vi "sendErrorExplanation.vi"(8 "error in (no error)":errorcluster, 11 "TcpServerBase in":refnum<class "TcpServerBase.lvclass">) -> (0 "error out":errorcluster, 3 "TcpServerBase out":refnum<class "TcpServerBase.lvclass">)   [LabVIEW 2018, in "TcpServerBase.lvclass"]
doc: "Send a generic user event to the Component with the explanation of the error."
uses:
  TcpServerBase.lvclass
  TcpServerCmd/typedef/connStatusCluster.ctl
  <vilib>/Utility/error.llb/DialogType.ctl
  TcpServerBase.lvclass/TcpServerBase.ctl
  TcpServerCmd/TcpServerCmd.lvclass
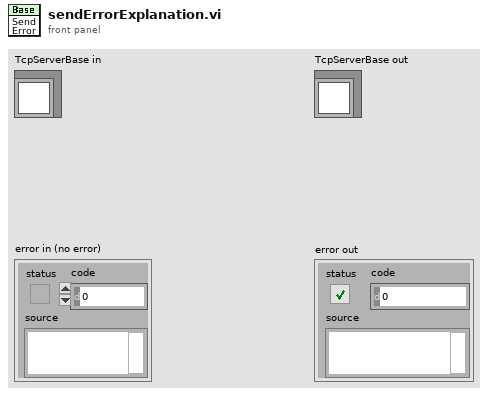
[diagram p1: front panel]
types:
  T1 = typedef "TcpServerCmd.lvclass/connStatusCluster.ctl" = cluster{"areClientsConnected":bool, "connStatusMsg":string}
  T2 = typedef "DialogType.ctl" = u16
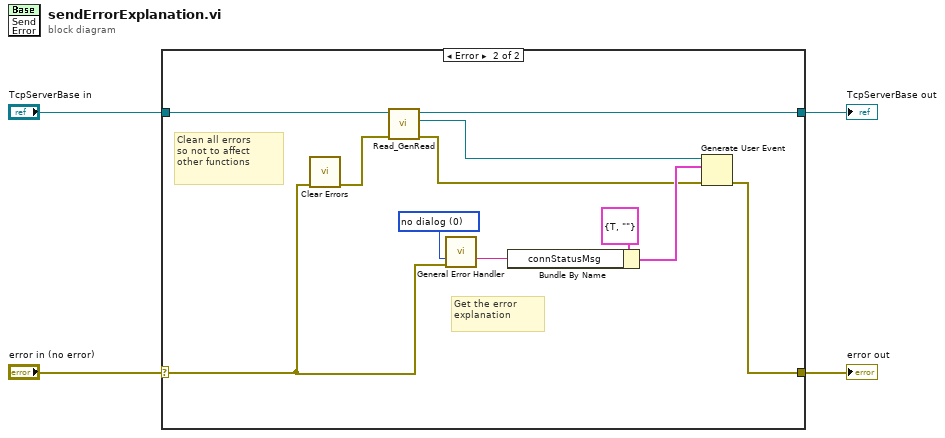
[diagram p0: block diagram]
diagram:
  n1 = case shown="Error" "error in (no error)" {
    selector: "error in (no error)" -> [w5 w8]
    tunnel: [w5 w15] -> w4
    tunnel: "TcpServerBase in" -> [w6 w12]
    tunnel: [w6 w11] -> w2
    frame No Error {
    }
    frame Error {
      w14 = T2 0 items=["no dialog", "OK message", "continue or stop message", "OK message + warnings", "continue/stop + warnings"] ("type of dialog (OK msg:1)")
      # "Clean all errors\nso not to affect\nother functions"
      # "Get the error\nexplanation"
      n2 = call <vilib>:"Clear Errors.vi"("error in (no error)"=w8) -> ("error out"=w10:errorcluster)  [unwired: 5 in, 1 out]
      n3 = call "Read_GenRead.vi"("error in (no error)"=w10, "TcpServerBase in"=w12) -> ("error out"=w9:errorcluster, "GenRead"=w7:refnum<user-event>, "TcpServerBase out"=w11:refnum<class "TcpServerBase.lvclass">)  [unwired: 7 in]
      n4 = call <vilib>:"General Error Handler.vi"("type of dialog (OK msg:1)"=w14, "error in (no error)"=w8) -> ("message"=w13:string)  [unwired: 9 in, 4 out]
      n5 = Bundle By Name(cluster=T1 {"areClientsConnected"=TRUE, "connStatusMsg"=""} ("event data"), "connStatusMsg"=w13) -> (w16:T1)
      n6 = Generate User Event(user event=w7, event data cluster=w16, error in=w9) -> (error out=w15:errorcluster)  [unwired: 1 in, 1 out]
    }
  }
  "TcpServerBase out" <- w2
  "error out" <- w4
